vi "NR_SourceData.vi"(0 "appended path":path, 1 "ParametersCluster":T1={"Nl"=1.0, "subframe_type"=1.0, "cp_type"=0.0, "cfi"=1.0, "UL_subframe_num"=2.0, "prb_num"=100.0, "module_type"=enum."64QAM", "mimo_type"=1.0}, 3 "imagestxpath":path) -> (4 "info_data":dbl[](array[numeric]), 5 "imagessendpath":path, 6 "error IO":errorcluster)   [LabVIEW 2015]
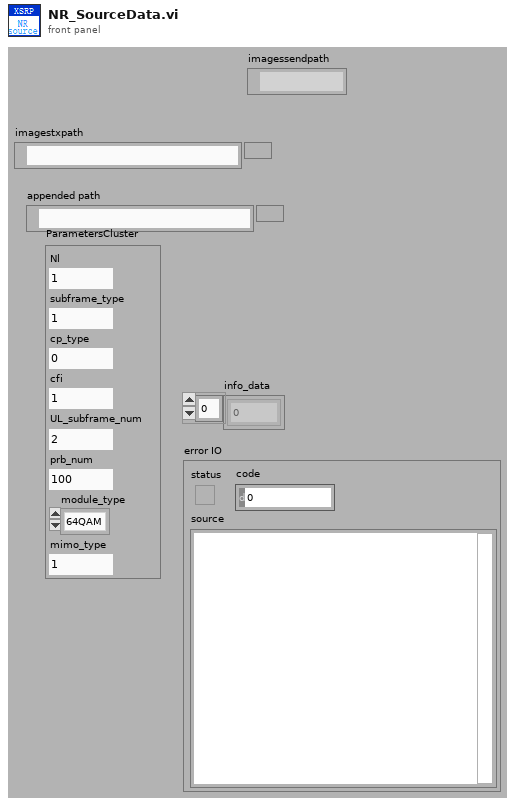
[diagram p1: front panel]
types:
  T1 = cluster{"Nl":dbl, "subframe_type":dbl, "cp_type":dbl, "cfi":dbl, "UL_subframe_num":dbl, "prb_num":dbl, "module_type":enum16{"", "QPSK", "16QAM", "64QAM", "256QAM"}, "mimo_type":dbl}
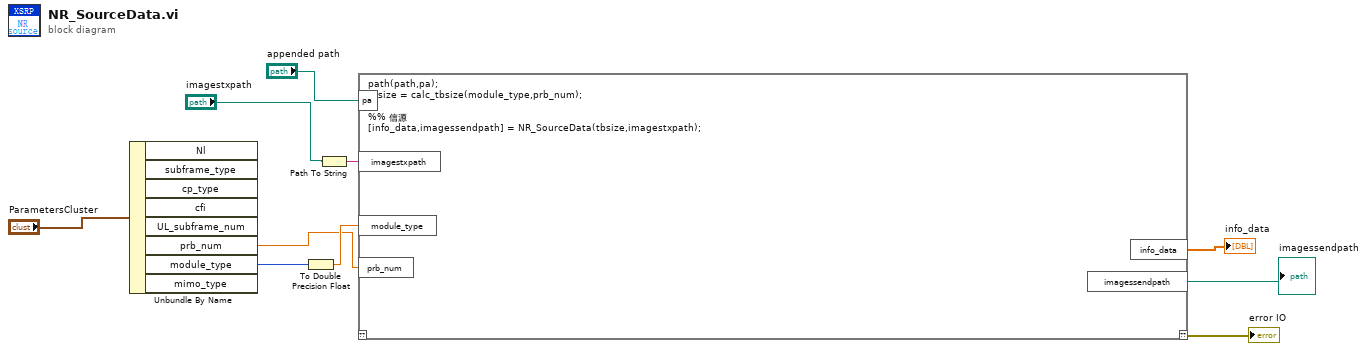
[diagram p0: block diagram]
diagram:
  n1 = Unbundle By Name("ParametersCluster") -> ("prb_num"=w4:dbl, "module_type"=w9:enum16{"", "QPSK", "16QAM", "64QAM", "256QAM"})  [unwired: 6 out]
  n2 = To Double Precision Float(number=w9) -> (double precision float=w5:dbl)
  n3 = Path To String(path="imagestxpath") -> (string=w2:string)
  n4 = script code="path(path,pa);\ntbsize = calc_tbsize(module_type,prb_num);\n\n%% 信源\n[info_data,imagessendpath] = NR_SourceData(tbsize,imagestxpath);"("pa"="appended path", "module_type"=w5, "prb_num"=w4, "imagestxpath"=w2) -> ("??"=→"error IO":errorcluster, "info_data"=→"info_data":dbl[], "imagessendpath"=→"imagessendpath":path)  [unwired: 1 in]
